vi "Initialize Variable List.vi"(8 "error in (no error)":errorcluster, 10 "Variable URLs In":refnum<k21>[](array[refnum]), 11 "Value List Reference In":refnum<vi>) -> (0 "error out":errorcluster, 2 "Variable URLs Out":refnum<k21>[](array[refnum]), 3 "Value List Reference Out":refnum<vi>)   [LabVIEW 2024]
doc: "Initializes the variable list in the subsystem view."
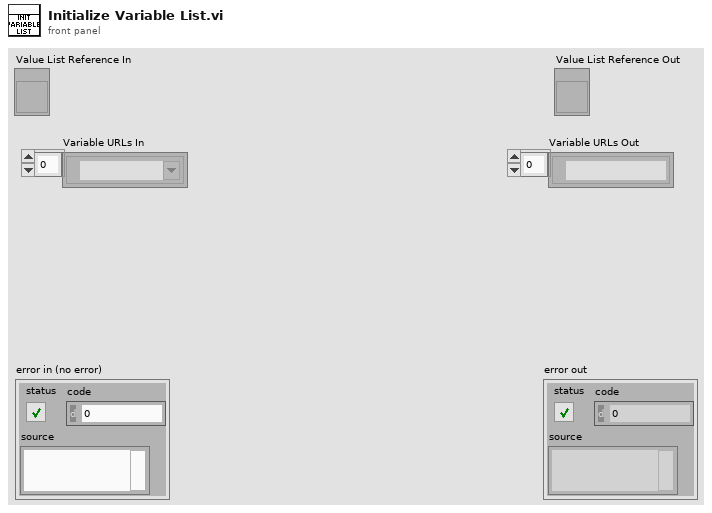
[diagram p1: front panel]
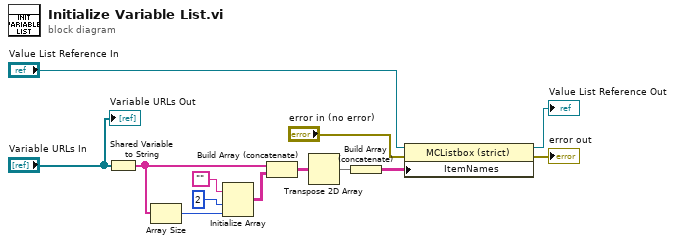
[diagram p0: block diagram]
diagram:
  n1 = Shared Variable to String(1:"Variable URLs In") -> (0:w3:string[])
  n2 = Array Size(array=w3) -> (size(s)=w4:i32)
  n3 = Initialize Array("", 2 ("dimension size"), w4) -> (w6:string[][])
  n4 = Build Array (concatenate)(w3, w6) -> (w5:string[][])
  n5 = Transpose 2D Array(2D array=w5) -> (transposed array=w8:string[][])
  n6 = Build Array (concatenate)(w8) -> (w1:string[][])
  n7 = property on="Property Node" class="MCListbox (strict)"(reference="Value List Reference In", error in="error in (no error)", "ItemNames"=w1) -> (reference out=→"Value List Reference Out":refnum<vi>, error out=→"error out":errorcluster)
  "Variable URLs Out" <- "Variable URLs In"
